vi "Unpack I32 Value.vi"(11 "I32ValueMsg in":refnum<class "I32ValueMsg.lvclass">) -> (2 "Value":i32, 3 "Name":string)   [LabVIEW 2015, in "ActorAutoRegistration.lvlib" / "I32ValueMsg.lvclass"]
uses:
  I32ValueMsg.lvclass
  I32ValueMsg.lvclass/I32ValueMsg.ctl
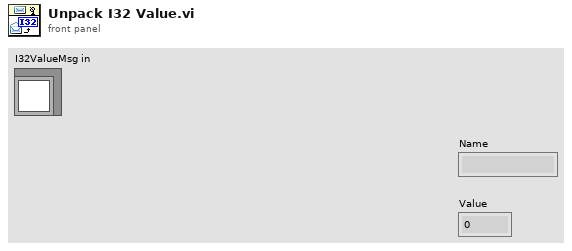
[diagram p1: front panel]
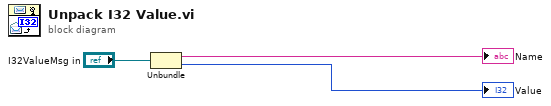
[diagram p0: block diagram]
diagram:
  n1 = Unbundle("I32ValueMsg in") -> (→"Name":string, →"Value":i32)
